vi "S2C_Shared_Func_Commands.vi"(8 "Error In":errorcluster, 9 "Settings":T1, 10 "Func-Q In":refnum<queue>, 11 "Proc-Q":refnum<queue>) -> (0 "Error Out":errorcluster, 1 "Timeout":dbl, 2 "Func-Q Out":refnum<queue>)   [LabVIEW 2015]
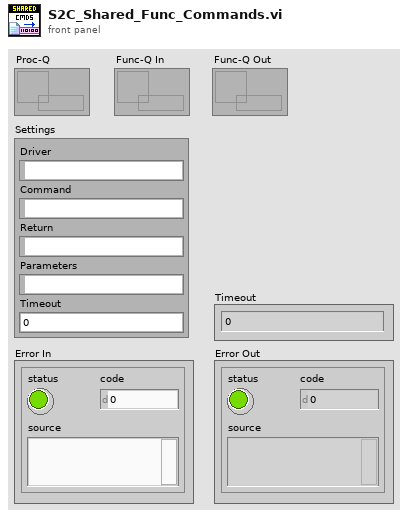
[diagram p1: front panel]
types:
  T1 = cluster{"Driver":string, "Command":string, "Return":string, "Parameters":string, "Timeout":dbl}
  T2 = cluster{"Caller-Q":refnum<queue>, "Command":string, "Return":string, "Data":variant, "Timeout":dbl}
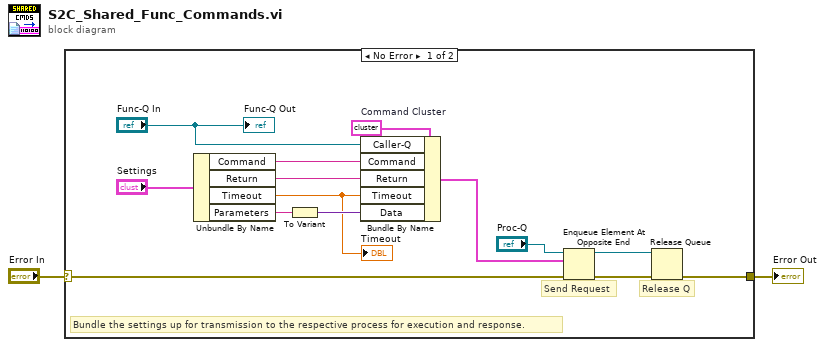
[diagram p0: block diagram]
diagram:
  n1 = case shown="No Error" "Error In" {
    selector: "Error In" -> [w11 w17]
    tunnel: [w13 w17] -> w1
    frame No Error {
      w4 = T2 {"Caller-Q"=refnum, "Command"="", "Return"="", "Data"=variant, "Timeout"=0.0}  # Command Cluster
      # "Bundle the settings up for transmission to the respective process for execution and response."
      # "Release Q"
      # "Send Request"
      n2 = Unbundle By Name("Settings") -> ("Command"=w9:string, "Return"=w8:string, "Timeout"=w5:dbl, "Parameters"=w7:string)
      "Timeout" <- w5
      n3 = To Variant(anything=w7) -> (Variant=w6:variant)
      n4 = Bundle By Name(cluster=w4, "Caller-Q"="Func-Q In", "Command"=w9, "Return"=w8, "Timeout"=w5, "Data"=w6) -> (w16:T2)
      n5 = Enqueue Element At Opposite End(queue="Proc-Q", element=w16, error in (no error)=w11) -> (queue out=w14:refnum<queue>, error out=w15:errorcluster)  [unwired: 1 in, 1 out]
      n6 = Release Queue(queue=w14, error in (no error)=w15) -> (error out=w13:errorcluster)  [unwired: 1 in, 2 out]
      "Func-Q Out" <- "Func-Q In"
    }
    frame Error {
    }
  }
  "Error Out" <- w1
